vi "TestVI_MonitoringPercentChange.vi"() -> ()   [LabVIEW 2026]
panel:
  out "x/y 2":dbl
  out "x/y":dbl
  out "Latest Samples":dbl[](array[numeric])
  in  "Array":dbl[](array[numeric])
  in  "stop":bool
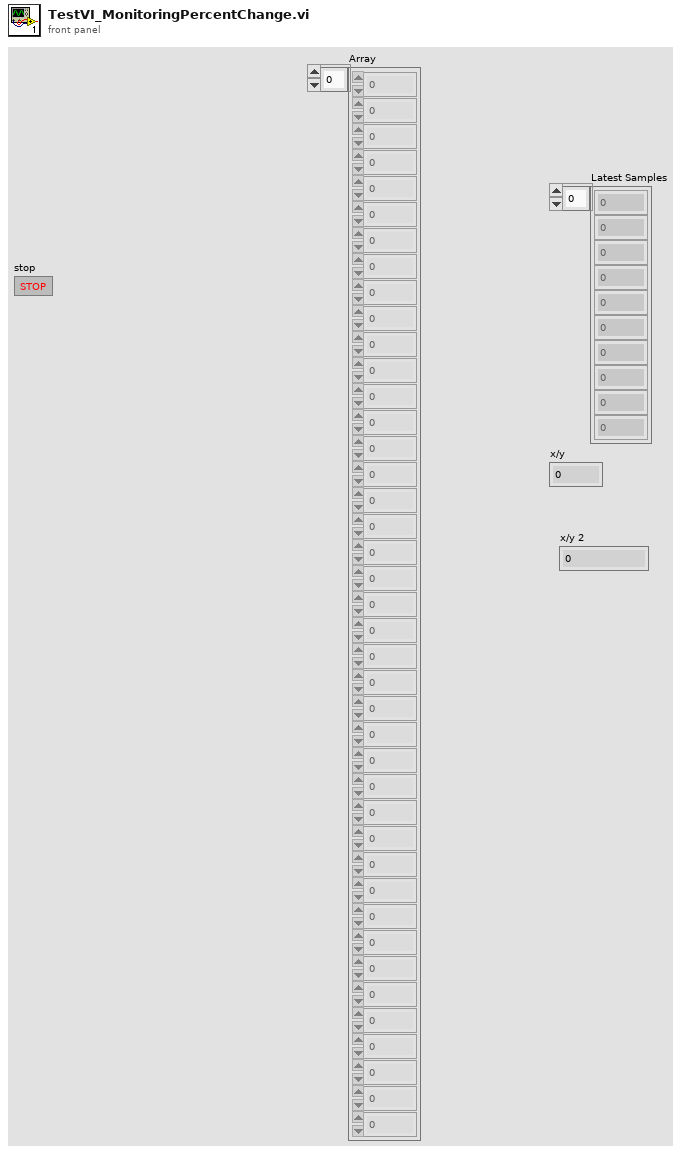
[diagram p1: front panel]
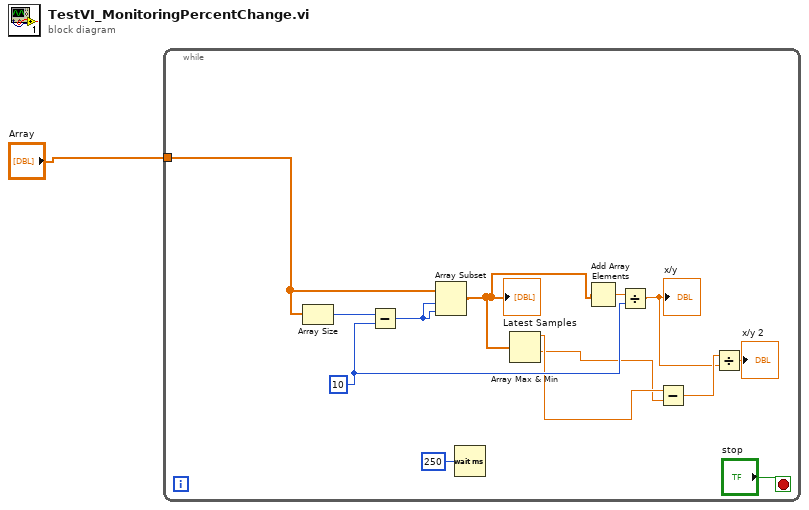
[diagram p0: block diagram]
diagram:
  n1 = while {
    tunnel: "Array" -> [w11]
    stop <- "stop" stop-if-true
    w7 = 10 ("y")
    n2 = Array Size(array=w11) -> (size(s)=w10:i32)
    n3 = Subtract(x=w10, y=w7) -> (x-y=w12:i32)
    n4 = Array Subset(array=w11, index=w12, length=w12) -> (w9:dbl[])
    "Latest Samples" <- w9
    n5 = Wait (ms)(milliseconds to wait=u32 250) -> ()  [unwired: 1 out]
    n6 = Array Max & Min(array=w9) -> (max value=w6:dbl, min value=w5:dbl)  [unwired: 2 out]
    n7 = Add Array Elements(numeric array=w9) -> (sum=w8:dbl)
    n8 = Divide(x=w8, y=w7) -> (x/y=w3:dbl)
    "x/y" <- w3
    n9 = Subtract(x=w6, y=w5) -> (x-y=w4:dbl)
    n10 = Divide(x=w4, y=w3) -> (x/y=→"x/y 2":dbl)
  }
